vi "Main.vi"   [LabVIEW 2018, in "Builder Pattern Demo.lvclass"]
uses:
  Builder Pattern Demo.lvclass
  Meal Builder Class/MealBuilder.lvclass
  ConsoleOut/Print Options.ctl
  Meal Class/Meal.lvclass
types:
  T1 = typedef "Print Options.ctl" = enum16{"Create", "Get Reference", "Print", "Print Header", "Close"}
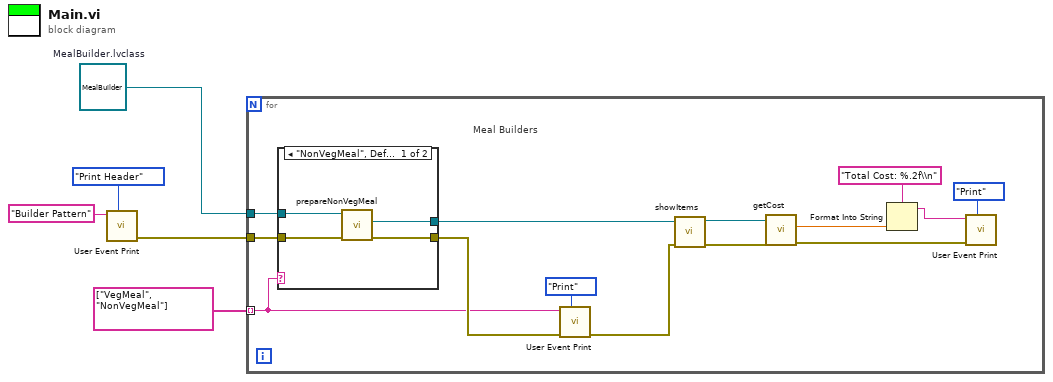
[diagram p0: block diagram]
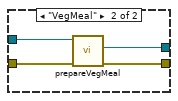
[diagram p2: hidden frame]
diagram:
  w5 = refnum<class "MealBuilder.lvclass"> refnum  # MealBuilder.lvclass
  n1 = call "User Event Print.vi"("Options"=Print_Options."Print Header", "String to Print"="Builder Pattern" ("message")) -> ("error out"=w3:errorcluster)  [unwired: 8 in, 1 out]
  n2 = for {
    tunnel: w5 -> [w14]
    tunnel: w3 -> [w7]
    tunnel: string[] ["VegMeal", "NonVegMeal"] ("message") -> [w6] mode=indexing
    # "Meal Builders"
    n3 = case shown="\"NonVegMeal\", Default" w6 {
      tunnel: [w23 w27] -> w17
      tunnel: w14 -> [w20 w26]
      tunnel: [w21 w25] -> w13
      tunnel: w7 -> [w22 w24]
      frame "NonVegMeal", Default {
        n4 = call-dynamic "prepareNonVegMeal.vi"("error in (no error)"=w22, "MealBuilder in"=w20) -> ("error out"=w23:errorcluster, "Meal out"=w21:refnum<class "Meal.lvclass">)  [unwired: 7 in, 1 out]
      }
      frame "VegMeal" {
        n5 = call-dynamic "prepareVegMeal.vi"("error in (no error)"=w24, "MealBuilder in"=w26) -> ("error out"=w27:errorcluster, "Meal out"=w25:refnum<class "Meal.lvclass">)  [unwired: 7 in, 1 out]
      }
    }
    n6 = call "User Event Print.vi"("Options"=Print_Options."Print", "error in (no error)"=w17, "String to Print"=w6) -> ("error out"=w12:errorcluster)  [unwired: 7 in, 1 out]
    n7 = call-dynamic "showItems.vi"("error in (no error)"=w12, "Meal in"=w13) -> ("error out"=w16:errorcluster, "Meal out"=w19:refnum<class "Meal.lvclass">)  [unwired: 8 in]
    n8 = call-dynamic "getCost.vi"("error in (no error)"=w16, "Meal in"=w19) -> ("error out"=w15:errorcluster, "cost"=w18:dbl)  [unwired: 7 in, 1 out]
    n9 = Format Into String(format string="Total Cost: %.2f\\n", w18) -> (resulting string=w9:string)  [unwired: 2 in, 1 out]
    n10 = call "User Event Print.vi"("Options"=Print_Options."Print", "error in (no error)"=w15, "String to Print"=w9) -> ()  [unwired: 7 in, 2 out]
  }
